vi "XY Graph Show-Hide Index Display Mask.vi"(8 "error in (no error)":errorcluster, 9 "Show(T)/Hide(F)":bool, 11 "XYGraph Ref":T1) -> (0 "error out":errorcluster, 1 "Found?":bool)   [LabVIEW 2021, in "XY Graph Add-Ons.lvlib"]
uses:
  XY Graph Add-Ons.lvlib
  XY Graph Refnum.ctl
  Utilities/Utilities.lvlib
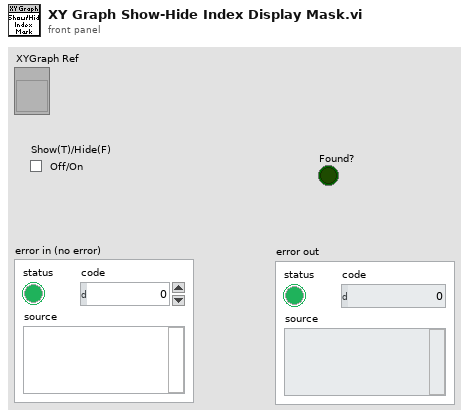
[diagram p1: front panel]
types:
  T1 = typedef "XY Graph Add-Ons.lvlib/XY Graph Refnum.ctl" = refnum<vi>
  T2 = enum16{"Controls & Indicators", "Controls", "Indicators"}
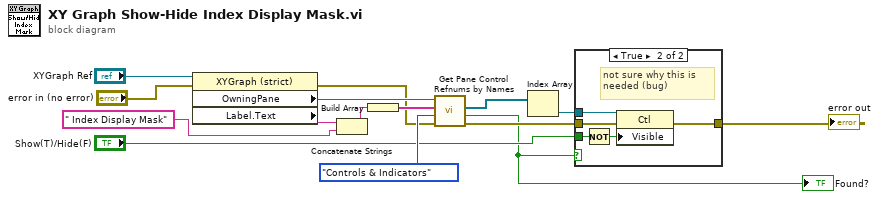
[diagram p0: block diagram]
diagram:
  n1 = property class="XYGraph (strict)"(reference="XYGraph Ref", error in="error in (no error)") -> (error out=w8:errorcluster, "OwningPane"=w10:refnum<vi>, "Label.Text"=w4:string)  [unwired: 1 out]
  n2 = Concatenate Strings(w4, " Index Display Mask" ("string")) -> (w14:string)
  n3 = Build Array(w14) -> (w13:string[])
  n4 = call "Get Pane Control Refnums by Names.vi"("error in"=w8, "Selection"=T2."Controls & Indicators", "Control Labels"=w13, "Pane Refnum"=w10) -> ("error out"=w6:errorcluster, "All Ctls found?"=w1:bool, "Ctl Refnums"=w11:refnum<vi>[])  [unwired: 5 in]
  "Found?" <- w1
  n5 = Index Array(array=w11) -> (element=w7:refnum<vi>)  [unwired: 1 in]
  n6 = case shown="True" w1 {
    tunnel: w7 -> [_ w21]
    tunnel: w6 -> [w16 w20]
    tunnel: [w16 w19] -> w5
    tunnel: "Show(T)/Hide(F)" -> [_ w18]
    frame False {
    }
    frame True {
      # "not sure why this is needed (bug)"
      n7 = Not(x=w18) -> (.not. x?=w17:bool)
      n8 = property class="Ctl"(reference=w21, error in=w20, "Visible"=w17) -> (error out=w19:errorcluster)  [unwired: 1 out]
    }
  }
  "error out" <- w5
